vi "Drive Controller.vi"(8 "error in":errorcluster) -> ()   [LabVIEW 2023]
doc: "This VI executes continuously carrying out the current operation and responding to updates or new operation requests. It will often contain the timing or control code that is difficult to place directly in TeleOp. This VI generally opens all sensors and motors and isolates the rest of the robot code from knowing implementation details of how the operations are carried out."
uses:
  Drive Operations.ctl
  bordeaux-pathinator/Bordeaux/Types/Segment Type.ctl
  Drive Setpoints.ctl
  swerve/Type Definitions/Data/Robot Velocities.ctl
  <vilib>/Rock Robotics/WPI/ThirdParty/REV Robotics/REVLib/Typedef/Spark MAX Control Type.ctl
  <vilib>/Rock Robotics/WPI/DriverStation/WPI_DriverStationRobotMode2.ctl
  e7fadf63-5109-474c-80f5-604bef1b4eb3.vi
  80b923c8-6b82-42f9-a8cd-acddf0fa8107.vi
  Framework/Robot Global Data.vi
  <vilib>/Rock Robotics/Network Tables/NT Write String.vi
  <vilib>/Rock Robotics/Network Tables/NT Read Numeric Array.vi
  <vilib>/Rock Robotics/Network Tables/NT Read Number.vi
  <vilib>/Platform/TimedLoop/XDataNode/XDataNode.xnode
  <vilib>/Platform/TimedLoop/XDataNode/nitl_modes.ctl
  <vilib>/Platform/TimedLoop/XDataNode/XDNodeRunTimeDep.lvlib
  <vilib>/Platform/TimedLoop/XDataNode/wakeup.ctl
  <vilib>/Platform/TimedLoop/XDataNode/timing_clust.ctl
  <vilib>/ptbypt/NI_PtbyPt.lvlib
  <vilib>/Rock Robotics/WPI/ThirdParty/Phoenix-LabVIEW/Pigeon IMU/CTRE_PigeonIMU_GetYPR.vi
panel:
  in  "Y Setpoint":dbl=-1.5
  in  "Right PID Setpoint":dbl=0.545
  in  "Left PID Setpoint":dbl=-0.49
  in  "Freeze Align?":bool
  out "VMag Sum":dbl
  out "Enabled VMag":dbl[](graph)
  out "Sum Angle":dbl
  out "Sum Y":dbl
  out "Sum X":dbl
  out "Enabled Omega":dbl[](graph)=[-0.0]
  out "Enabled Y Velocity":dbl[](graph)
  out "Enabled X Velocity":dbl[](graph)
  out "Trajectory Velocity":dbl[](graph)
  out "Trajectory Data Compare":T2(array[cluster])
  out "Trajectory Data Out":T2(array[cluster])=[{"Segment Name"="Linear 0", "Type"=enum."Accel Straight", "Traj Pos Points"=[{"x"=-0.07702359916175033, "y"=-1.5597275539829196, "th"=0.3959786593914032}], "Traj Vel Points"=[{"V"=0.0, "Omega"=-0.0, "V vector"={"y"=-0.0, "x"=0.0}}], "Accel Index"=0, "Decel Index"=1}, {"Segment Name"="", "Type"=enum."Accel Straight", "Traj Pos Points"=[], "Traj Vel Points"=[], "Accel Index"=0, "Decel Index"=0}]
  in  "PID enabled":bool=TRUE
  out "Trapezoid Profile":dbl[](graph)
  out "Weird Aligning Code?":string
  in  "Go Up?":i32
  in  "Int per ft":dbl=0.75
  in  "PID gains":T3={"proportional gain (Kp)"=1.5, "integral time (Ki)"=0.075, "derivative time (Kd)"=0.0} {"derivative time (Kd)" format="%.3f"; "integral time (Ki)" format="%.3f"; "proportional gain (Kp)" format="%.3f"}
  out "PID Out":dbl=0.10498956284304024
  out "Waveform Chart":cluster{dbl, "Right X Setpoint":dbl}(graph)={-0.574331443611901, "Right X Setpoint"=-0.559167}
  in  "Operation":T4
  in  "Auto PID Constants":T5={"P Gain"=0.09, "I Gain"=0.0, "D Gain"=0.0, "F Gain"=0.08, "I Zone"=0.0, "Min Output"=-1.0, "Max Output"=1.0}
  in  "Immediate PID Constants":T5={"P Gain"=0.09, "I Gain"=0.0, "D Gain"=0.0, "F Gain"=0.08, "I Zone"=0.0, "Min Output"=-1.0, "Max Output"=1.0}
  out "Waveform Chart":cluster{"Numeric":dbl, "Numeric":dbl}(graph)
  in  "Period":i32=26
  in  "Acceleration Max":dbl=3.0
  in  "Velocity Max":dbl=6.0
  in  "Left X Setpoint":dbl=-0.609167
  in  "Left Y Setpoint":dbl
  in  "Right Y Setpoint":dbl
  in  "Right X Setpoint":dbl=0.559167
  in  "Deadband":T6={"Angle (deg)"=3.0, "X (ft)"=0.1, "Y (ft)"=0.125}
  in  "Drive Controller Diagnostics":T7(tab)
  out "Swerve Visualizer":cluster{dbl[], dbl[]}[](graph)
  out "Pod Comparisons (Diff -> Setpoint - Actual)":T8
  out "(Calibration) Steering Angles":T9={"Left Front"=134.8391571044922, "Left Back"=135.21200561523438, "Right Front"=135.20999145507812, "Right Back"=-44.576202392578125}
  out "Current\nCmd":string="Started at  21:02:15.312\nDefault: Reserve,  Vx 0.0, Vy 0.0, W 0.000000"
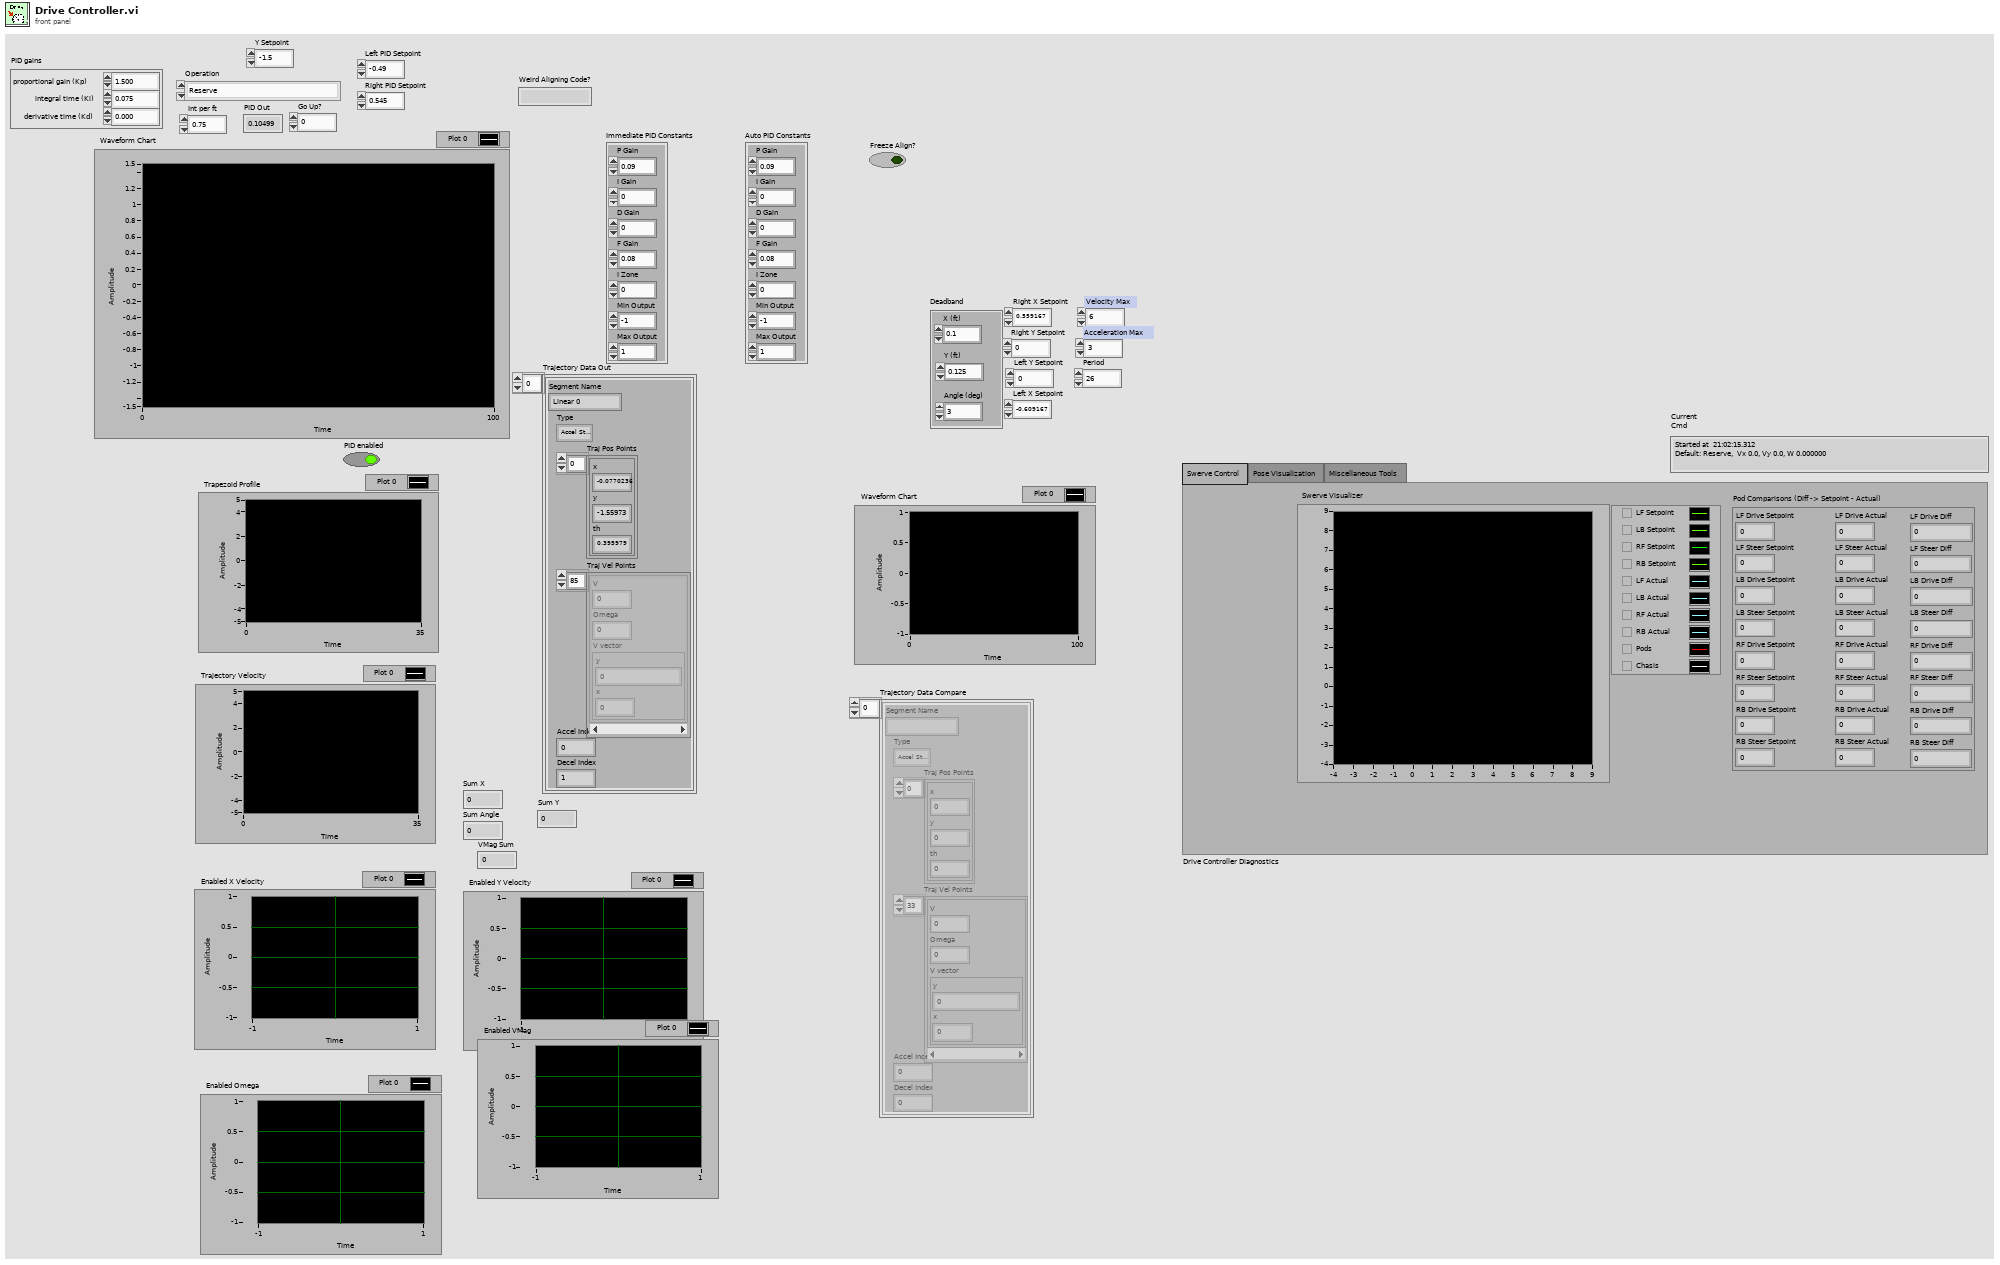
[diagram p1: front panel]
types:
  T1 = typedef "Segment Type.ctl" = enum16{"Accel Straight", "Const Straight", "Blend", "Circle", "Bezier"}
  T2 = cluster{"Segment Name":string, "Type":T1, "Traj Pos Points":cluster{"x":dbl, "y":dbl, "th":dbl}[], "Traj Vel Points":cluster{"V":dbl, "Omega":dbl, "V vector":cluster{"y":dbl, "x":dbl}}[], "Accel Index":i32, "Decel Index":i32}[]
  T3 = cluster{"proportional gain (Kp)":dbl, "integral time (Ki)":dbl, "derivative time (Kd)":dbl}
  T4 = typedef "Drive Operations.ctl" = enum16{"Reserve", "Read Current", "Immediate", "Calibrate", "Reef Align", "Auto"}
  T5 = cluster{"P Gain":dbl, "I Gain":dbl, "D Gain":dbl, "F Gain":dbl, "I Zone":dbl, "Min Output":dbl, "Max Output":dbl}
  T6 = cluster{"Angle (deg)":dbl, "X (ft)":dbl, "Y (ft)":dbl}
  T7 = enum32{"Swerve Control", "Pose Visualization", "Miscellaneous Tools"}
  T8 = cluster{"LF Drive Setpoint":dbl, "LF Steer Setpoint":dbl, "LB Drive Setpoint":dbl, "LB Steer Setpoint":dbl, "RF Drive Setpoint":dbl, "RF Steer Setpoint":dbl, "RB Drive Setpoint":dbl, "RB Steer Setpoint":dbl, "LF Drive Actual":dbl, "LF Steer Actual":dbl, "LB Drive Actual":dbl, "LB Steer Actual":dbl, "RF Drive Actual":dbl, "RF Steer Actual":dbl, "RB Drive Actual":dbl, "RB Steer Actual":dbl, "LF Drive Diff":dbl, "LF Steer Diff":dbl, "LB Drive Diff":dbl, "LB Steer Diff":dbl, "RF Drive Diff":dbl, "RF Steer Diff":dbl, "RB Drive Diff":dbl, "RB Steer Diff":dbl}
  T9 = cluster{"Left Front":dbl, "Left Back":dbl, "Right Front":dbl, "Right Back":dbl}
  T10 = typedef "Drive Setpoints.ctl" = cluster{"Operation":T4, "Robot Velocities":T11, "Auto Data":cluster{"Auto Velocities":T11[], "Auto Positions":cluster{"x":dbl, "y":dbl, "th":dbl}[], "Auto Commands":cluster{dbl, "Command out":cluster{"Name":string, "vi reference":refnum<vi>, i32[], variant[]}}[], "Zero Velocity?":bool[]}, "Left side":bool, "Angle Align":bool, "Tag ID":i32}
  T11 = typedef "Robot Velocities.ctl" = cluster{"X Velocity":dbl, "Y Velocity":dbl, "Rotational \nVelocity":dbl}
  T12 = typedef "(NEO-NEO-ThroughBore-Pigeon2) Swerve.ctl" = cluster{"Drive Motors (NEO)":T13, "Steer Motors (NEO)":T13, "Pigeon2":T19, "Radii (ft)":T21}
  T13 = typedef "(NEO & NEO 550) 4 Motor Set.ctl" = cluster{"Left Front":T14, "Left Back":T14, "Right Front":T14, "Right Back":T14}
  T14 = typedef "WPI_MotorControlDeviceRef.ctl" = cluster{"DeviceStatus":errorcluster, "Type":T15, "PWM":cluster{"PWM Channel":T16, "DeadBand":T17}, "CAN":cluster{"Device Number":u8, "SetOutput VI Ref":variant, "GetOutput VI Ref":variant, "Enable VI Ref":variant, "Disable VI Ref":variant, "Data":variant}, "Invert":bool, "DIO PWM":cluster{"PWM \"Enable\" Channel":T16, "DIOChannel":T18, "PWM Rate":dbl}}
  T15 = typedef "WPI_MotorControlType.ctl" = enum16{"PWM", "CAN", "DIO PWM"}
  T16 = typedef "FPGA_DIOPWMChannel.ctl" = enum8{"PWM 0", "PWM 1", "PWM 2", "PWM 3", "PWM 4", "PWM 5", "PWM 6", "PWM 7", "PWM 8", "PWM 9", "PWM MXP 0", "PWM MXP 1", "PWM MXP 2", "PWM MXP 3", "PWM MXP 4", "PWM MXP 5", "PWM MXP 6", "PWM MXP 7", "PWM MXP 8", "PWM MXP 9", "Invalid"}
  T17 = typedef "WPI_PWMDeadband.ctl" = cluster{"Name":string, "maxPositivePwm":i32, "minPositivePwm":i32, "centerPwm":i32, "maxNegativePwm":i32, "minNegativePwm":i32, "angularRange":u16}
  T18 = typedef "FPGA_DIOChannel.ctl" = enum8{"DIO 0", "DIO 1", "DIO 2", "DIO 3", "DIO 4", "DIO 5", "DIO 6", "DIO 7", "DIO 8", "DIO 9", "DIO MXP 0", "DIO MXP 1", "DIO MXP 2", "DIO MXP 3", "DIO MXP 4", "DIO MXP 5", "DIO MXP 6", "DIO MXP 7", "DIO MXP 8", "DIO MXP 9", "DIO MXP 10", "DIO MXP 11", "DIO MXP 12", "DIO MXP 13", "DIO MXP 14", "DIO MXP 15", "SPI Port CS1", "SPI Port CS2", "SPI Port CS3", "SPI Port MISO", "SPI Port MOSI", "Invalid"}
  T19 = typedef "CTRE_PigeonIMU_DeviceRef.ctl" = cluster{"DeviceStatus":errorcluster, "Device Number":u8, "Type":T20, "Device ID":u32, "Handle":u64, "UsageFrame":u32, "Library Path":path}
  T20 = typedef "CTRE_PigeonIMU_ConnectionType.ctl" = u32
  T21 = typedef "Pod Positions.ctl" = cluster{"Left Front Position":dbl[], "Left Back Position":dbl[], "Right Front Position":dbl[], "Right Back Position":dbl[]}
  T22 = typedef "Command Status Info.ctl" = cluster{"Name":string, "Status":T23, "notifier out":T24}
  T23 = typedef "Completion Status.ctl" = enum16{"Successful", "Aborted", "Incomplete"}
  T24 = typedef "Completion Notifier.ctl" = refnum<notifier>
  T25 = cluster{"SubSystem Data":T10, cluster{"Start Time (ms)":u32, "Iterations":i32}, cluster{"Command Info":T22, "Description":string, "Default Command":T10, "queue out":refnum<queue>, "Subsystem Name":string}}
  T26 = typedef "Spark MAX Control Type.ctl" = enum16{"Percent VBus", "Voltage", "Velocity", "Position", "Smart Motion", "Current", "Smart Velocity", "MAXMotion Position", "MAXMotion Velocity"}
  T27 = typedef "WPI_DriverStationRobotMode2.ctl" = enum16{"Autonomous Disabled", "Autonomous Enabled", "Teleop Disabled", "Teleop Enabled", "Disconnected", "Finish", "Test Disabled", "Test Enabled", "Emergency Stopped"}
  T28 = typedef "XDNodeRunTimeDep.lvlib/timing_clust.ctl" = cluster{"Expected End [f-1]":u64, "Actual End [f-1]":u64, "Finished Late? [f-1]":bool, "Expected End [i-1]":u64, "Actual End [i-1]":u64, "Finished Late? [i-1]":bool, "Expected Start [i]":u64, "Actual Start [i]":u64, "Expected Start [f]":u64, "Actual Start [f]":u64, "Source Name":string, "Structure Name":string, "Period":i64, "Deadline":i64, "Offset":i64, "Start":i64, "Priority":i32, "Timeout":i32, "Mode":T29, "Wakeup Reason":T30, "Error":errorcluster, "Source Type":string, "Secondary Source Type":string, "Global End Time":u64, "Global Start Time":u64, "Frame Duration":u64, "Iteration Duration":u64, "Assigned CPU":i32, "I/O Scan Engine Mode":u32}
  T29 = typedef "XDNodeRunTimeDep.lvlib/nitl_modes.ctl" = enum32{"No Change", "Process missed periods, maintain original phase", "Discard missed periods, maintain original phase", "Process missed periods, ignore original phase", "Discard missed periods, ignore original phase"}
  T30 = typedef "XDNodeRunTimeDep.lvlib/wakeup.ctl" = enum32{"Normal", "Aborted", "Asynchronous wakeup", "Timing source error", "Timed loop error", "Timeout"}
  T31 = cluster{"Auto Velocities":T11[], "Auto Positions":cluster{"x":dbl, "y":dbl, "th":dbl}[], "Auto Commands":cluster{dbl, "Command out":cluster{"Name":string, "vi reference":refnum<vi>, i32[], variant[]}}[], "Zero Velocity?":bool[]}
  T32 = cluster{"Field Centric":bool, "Reef Centric":bool}
  T33 = typedef "Pod Setpoints.ctl" = cluster{"Left Front":cluster{"Velocity":dbl, "Theta":dbl}, "Left Back":cluster{"Velocity":dbl, "Theta":dbl}, "Right Front":cluster{"Velocity":dbl, "Theta":dbl}, "Right Back":cluster{"Velocity":dbl, "Theta":dbl}}
  T34 = cluster{"Left X Setpoint":dbl, "Left Y Setpoint":dbl}
  T35 = cluster{"Right X Setpoint":dbl, "Right Y Setpoint":dbl}
  T36 = cluster{"Segment Name":string, "Type":T1, "Traj Pos Points":cluster{"x":dbl, "y":dbl, "th":dbl}[], "Traj Vel Points":cluster{"V":dbl, "Omega":dbl, "V vector":cluster{"y":dbl, "x":dbl}}[], "Accel Index":i32, "Decel Index":i32}
  T37 = cluster{"V":dbl, "Omega":dbl, "V vector":cluster{"y":dbl, "x":dbl}}[]
  T38 = cluster{"Filtered x":dbl, "Right X Setpoint":dbl}
  T39 = cluster{"Right X Setpoint":dbl, "Y Setpoint":dbl, dbl}
  T40 = cluster{"SubSystem Data":T10, cluster{"Start Time (ms)":u32, "Iterations":i32}, "Default Command Arguments":cluster{"Command Info":T22, "Description":string, "Default Command":T10, "queue out":refnum<queue>, "Subsystem Name":string}}
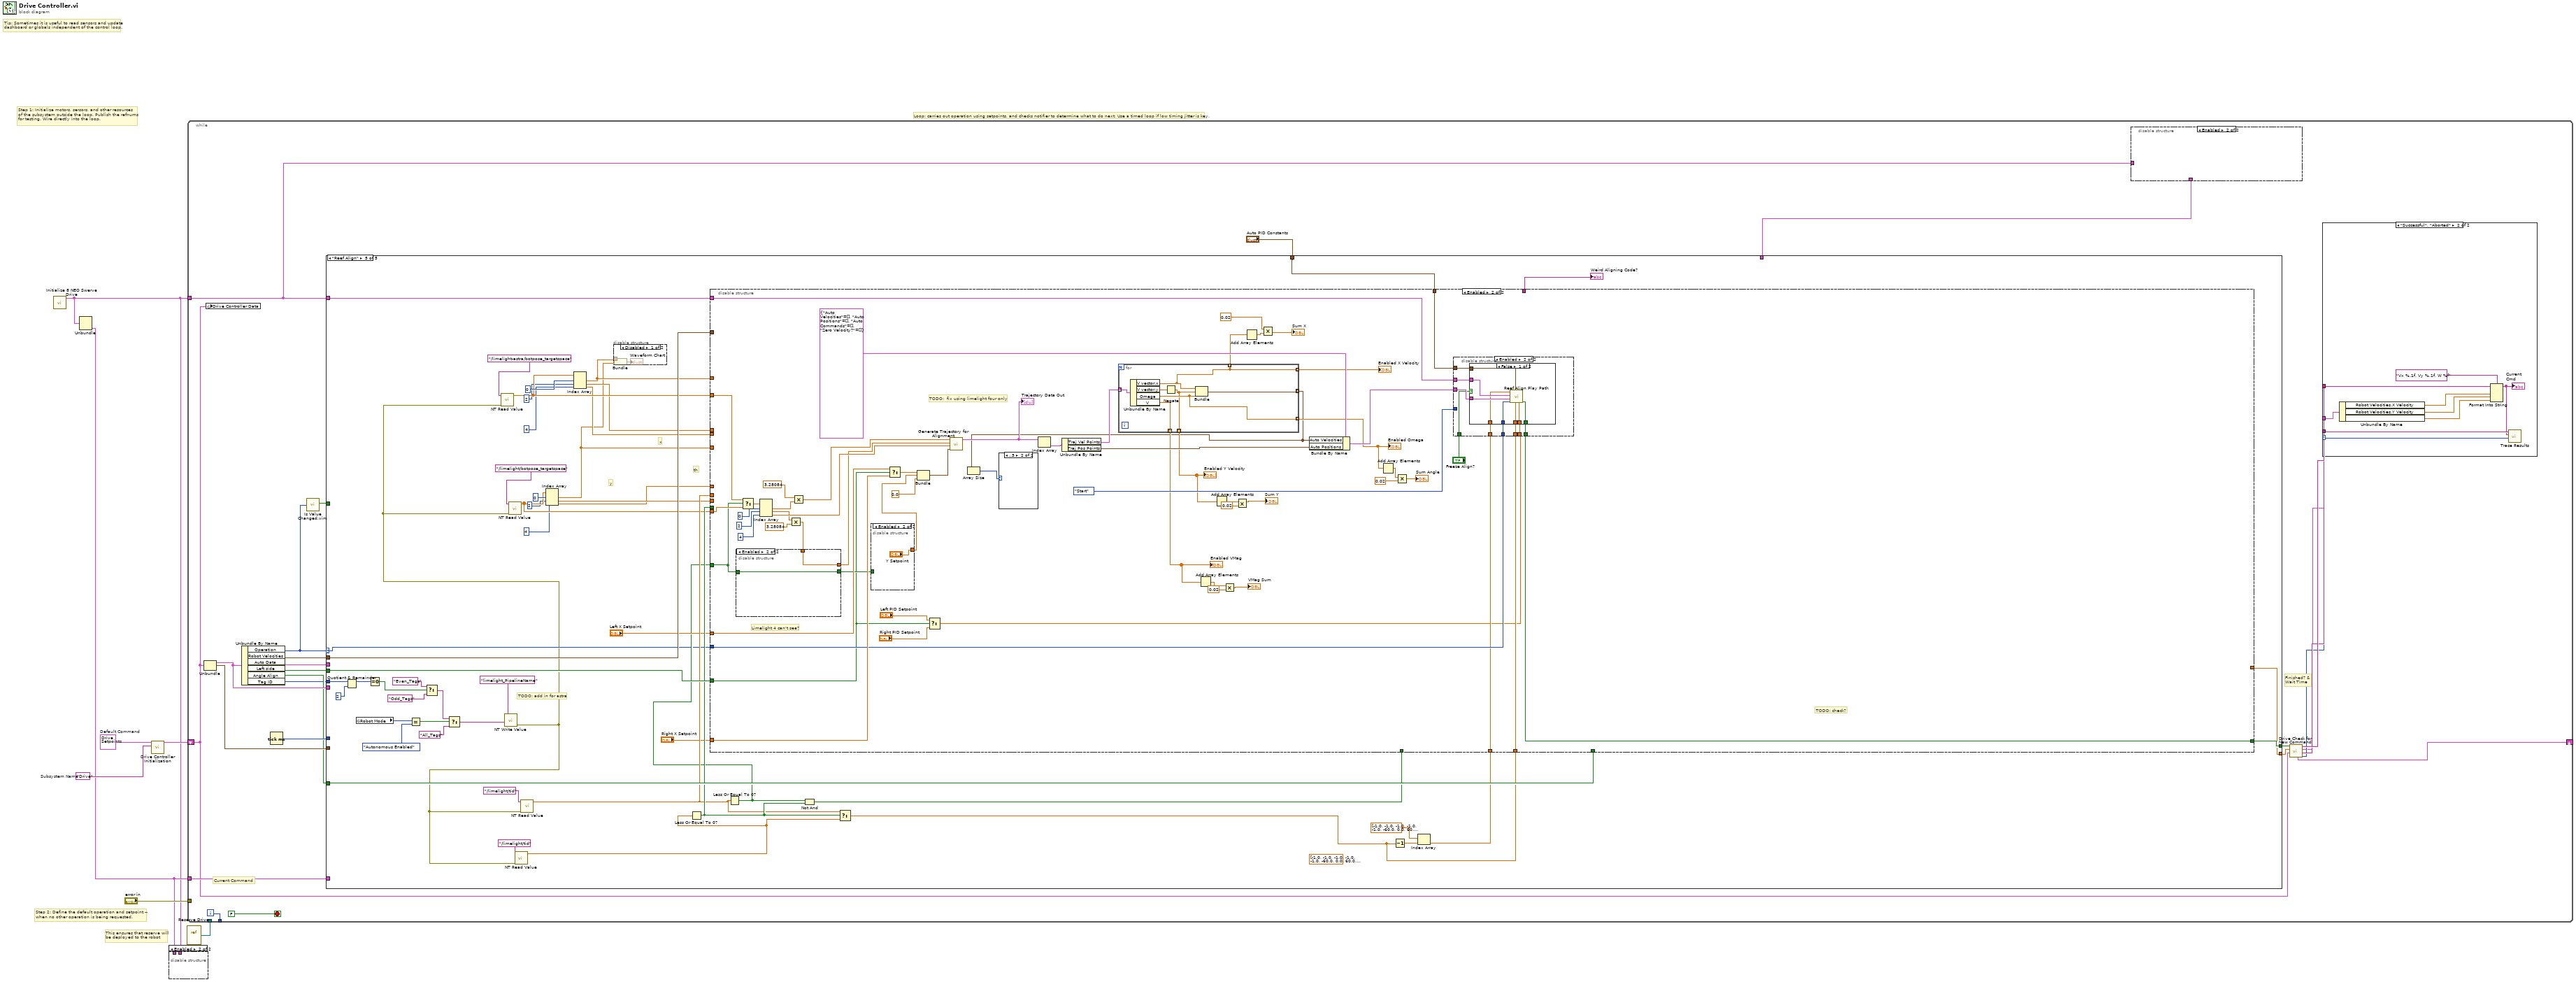
[diagram p0: block diagram]
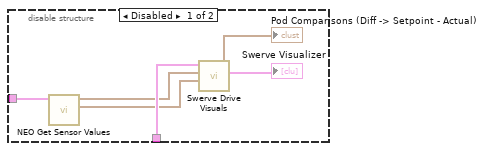
[diagram p2: hidden frame]
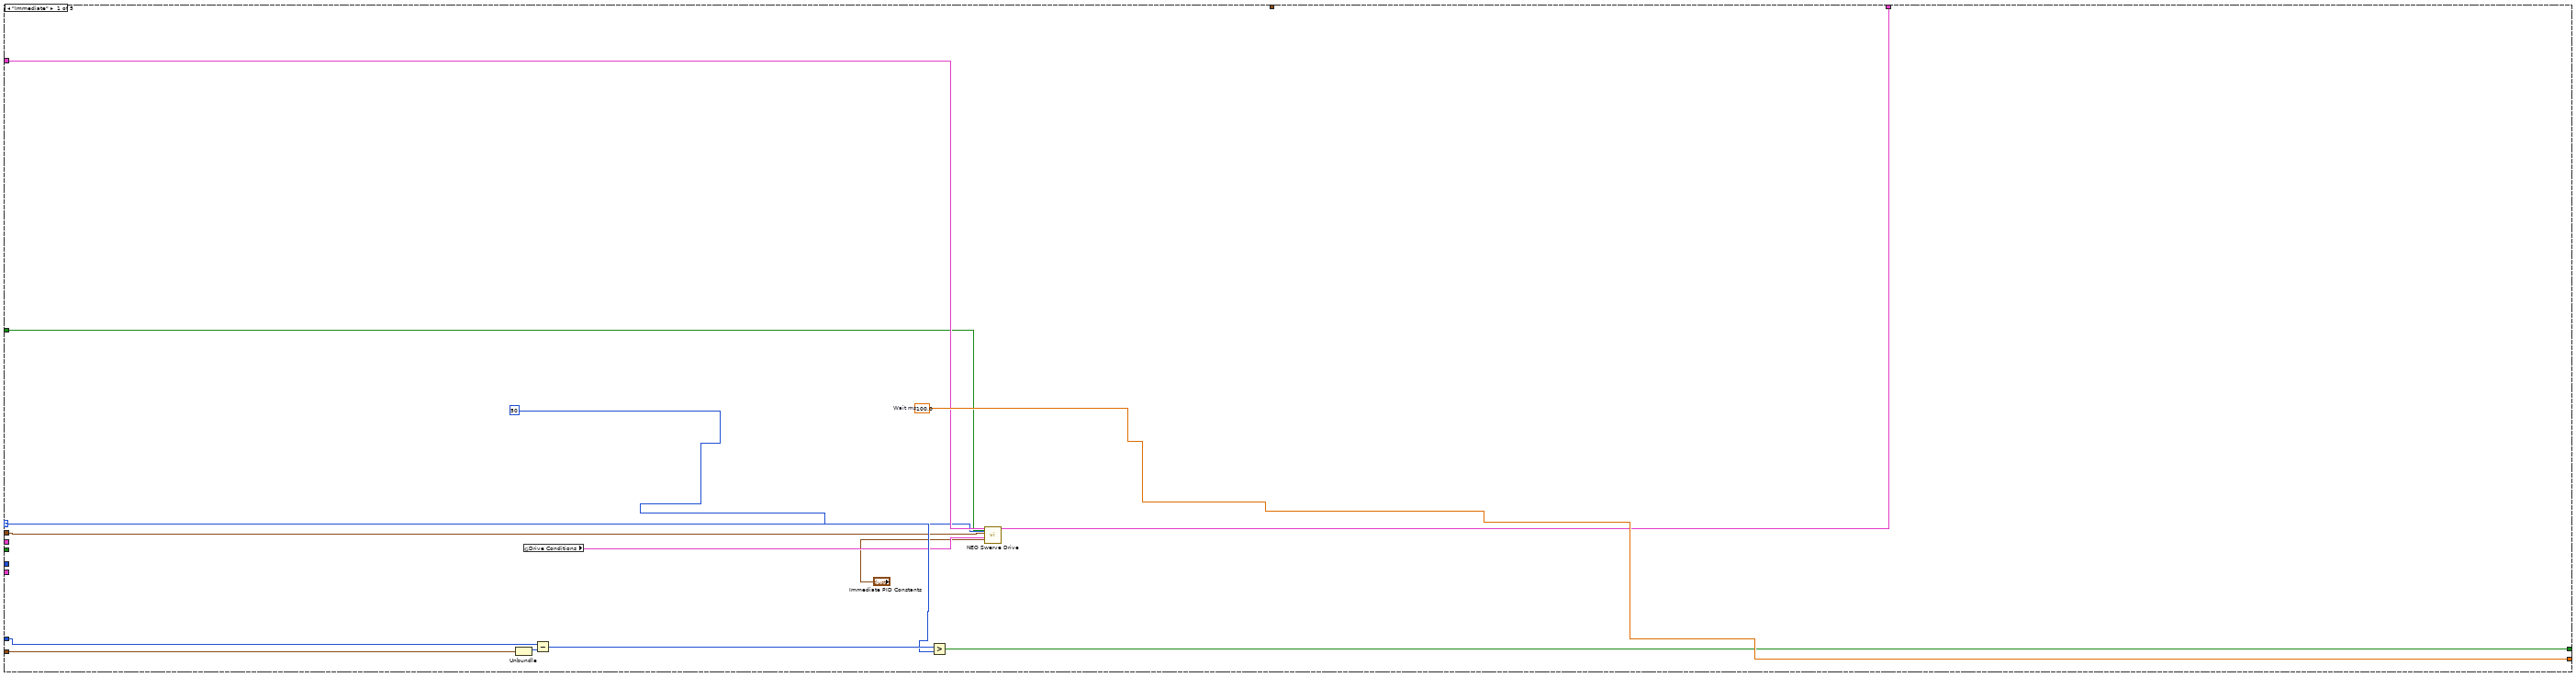
[diagram p3: hidden frame]
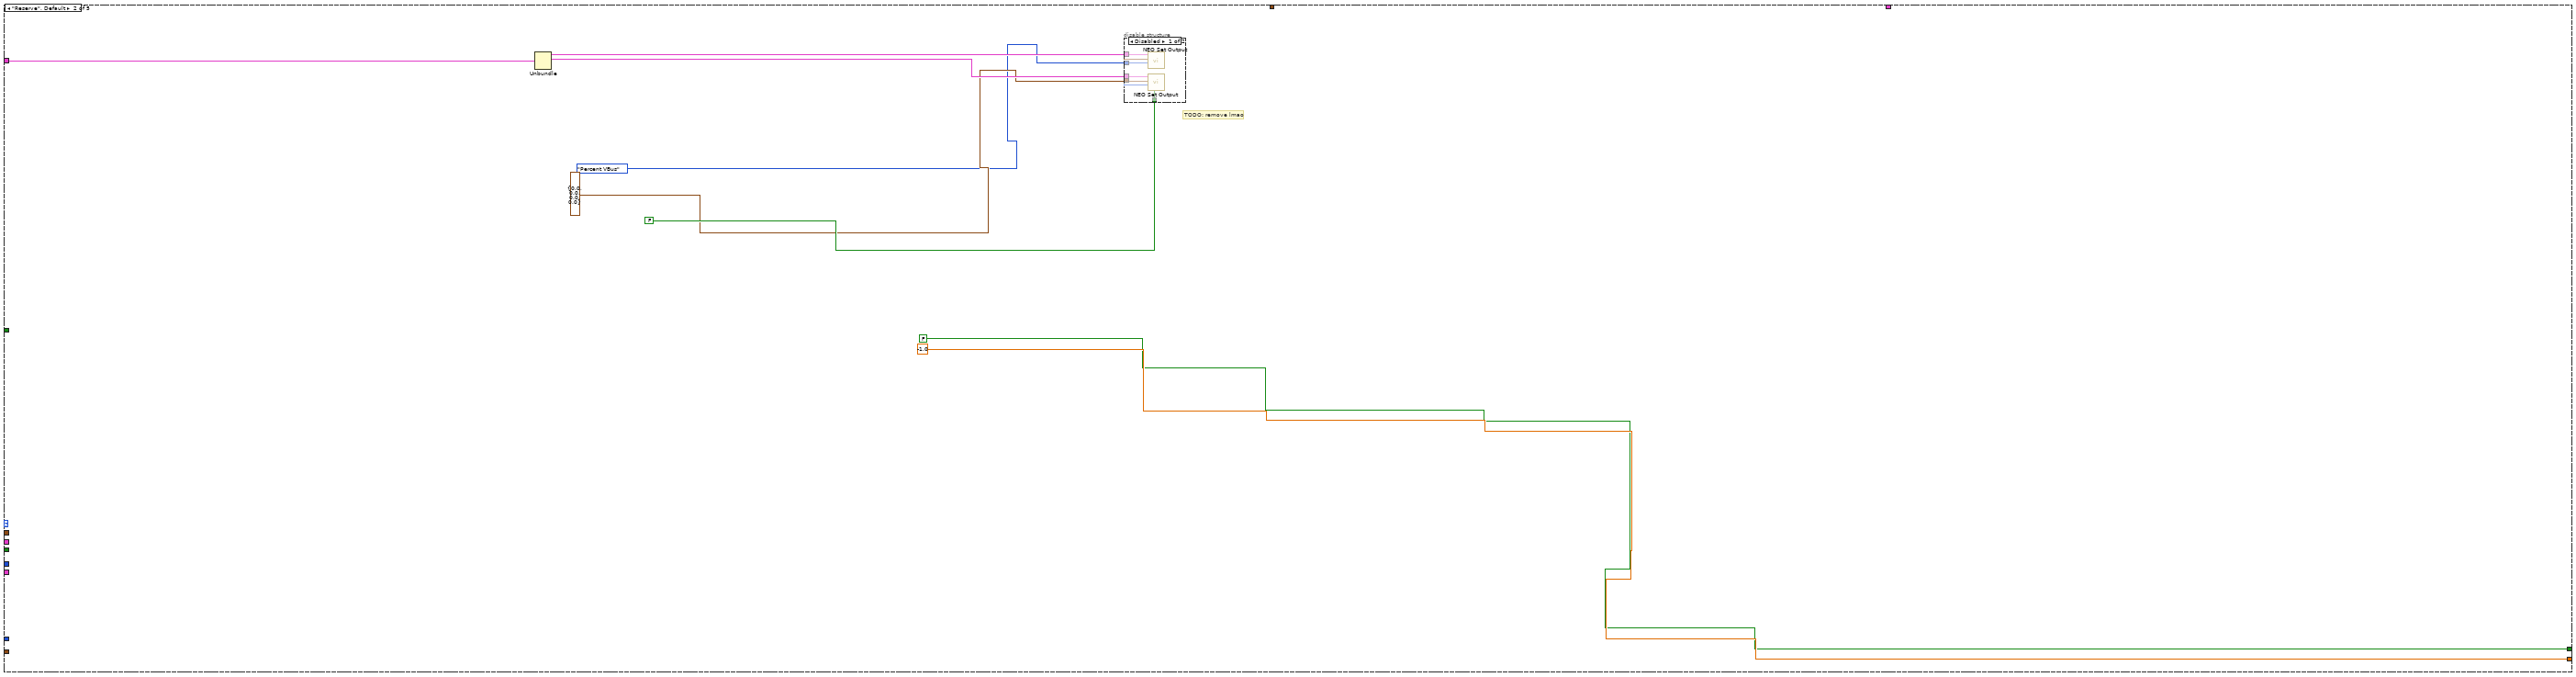
[diagram p4: hidden frame]
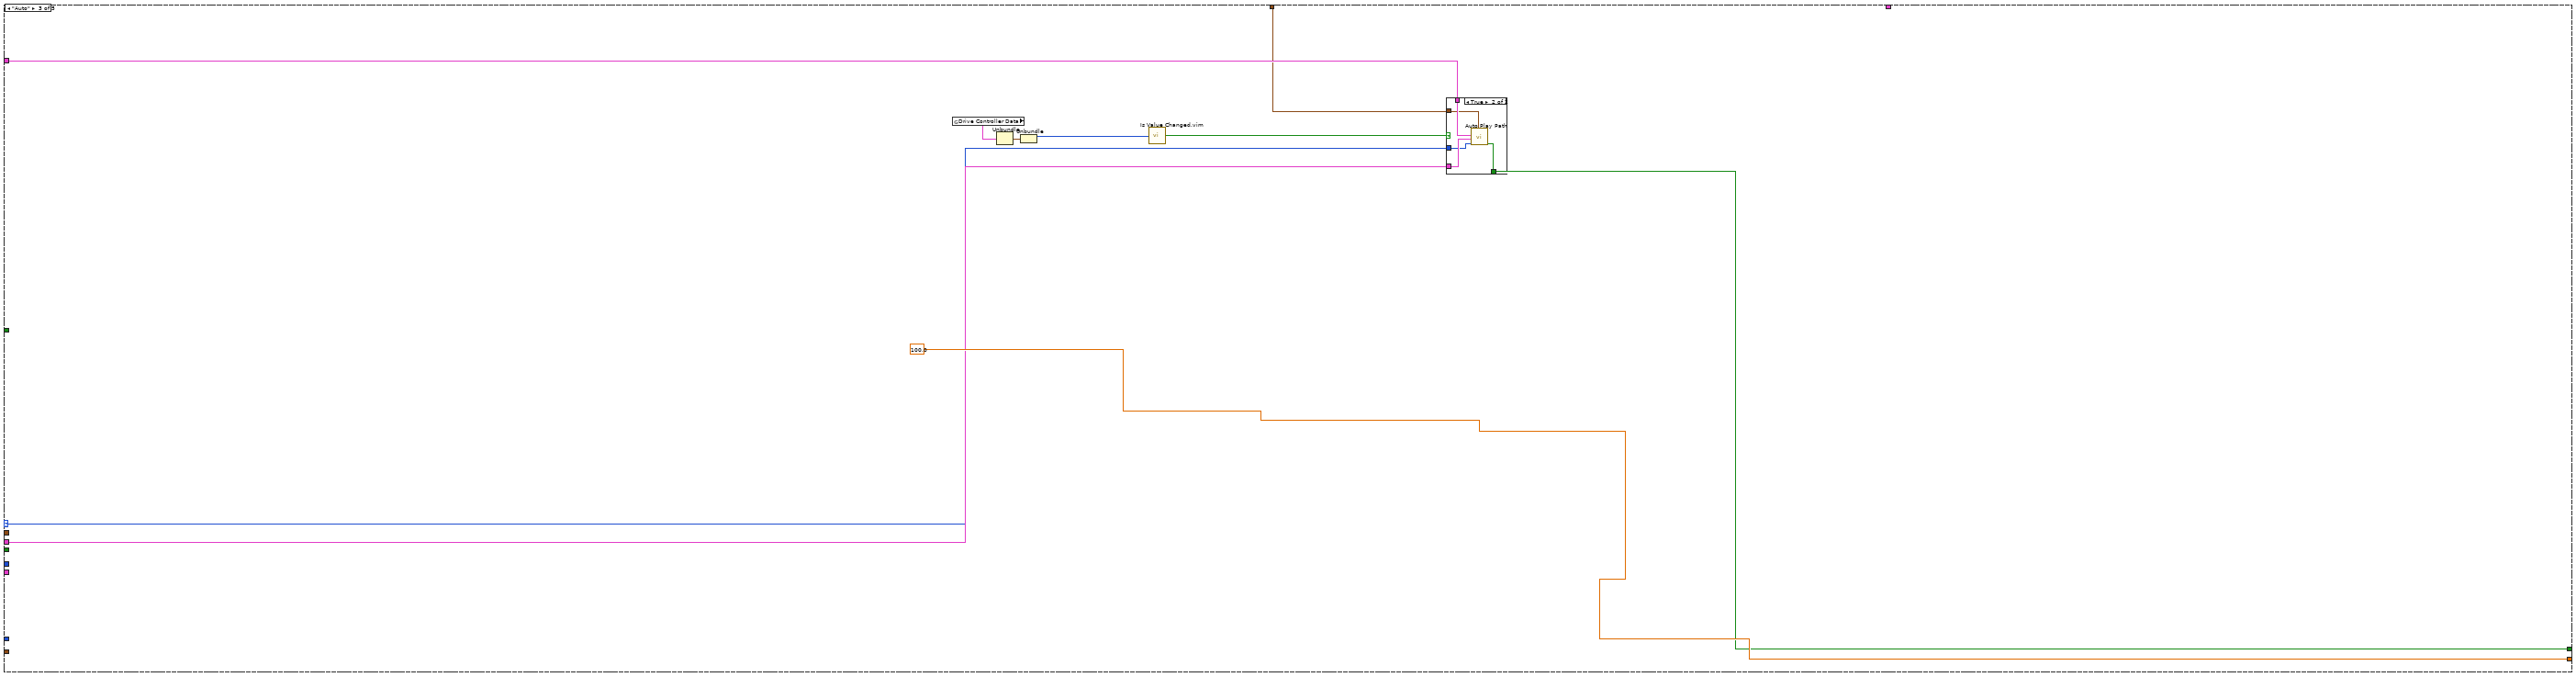
[diagram p6: hidden frame]
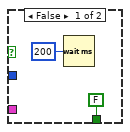
[diagram p7: hidden frame]
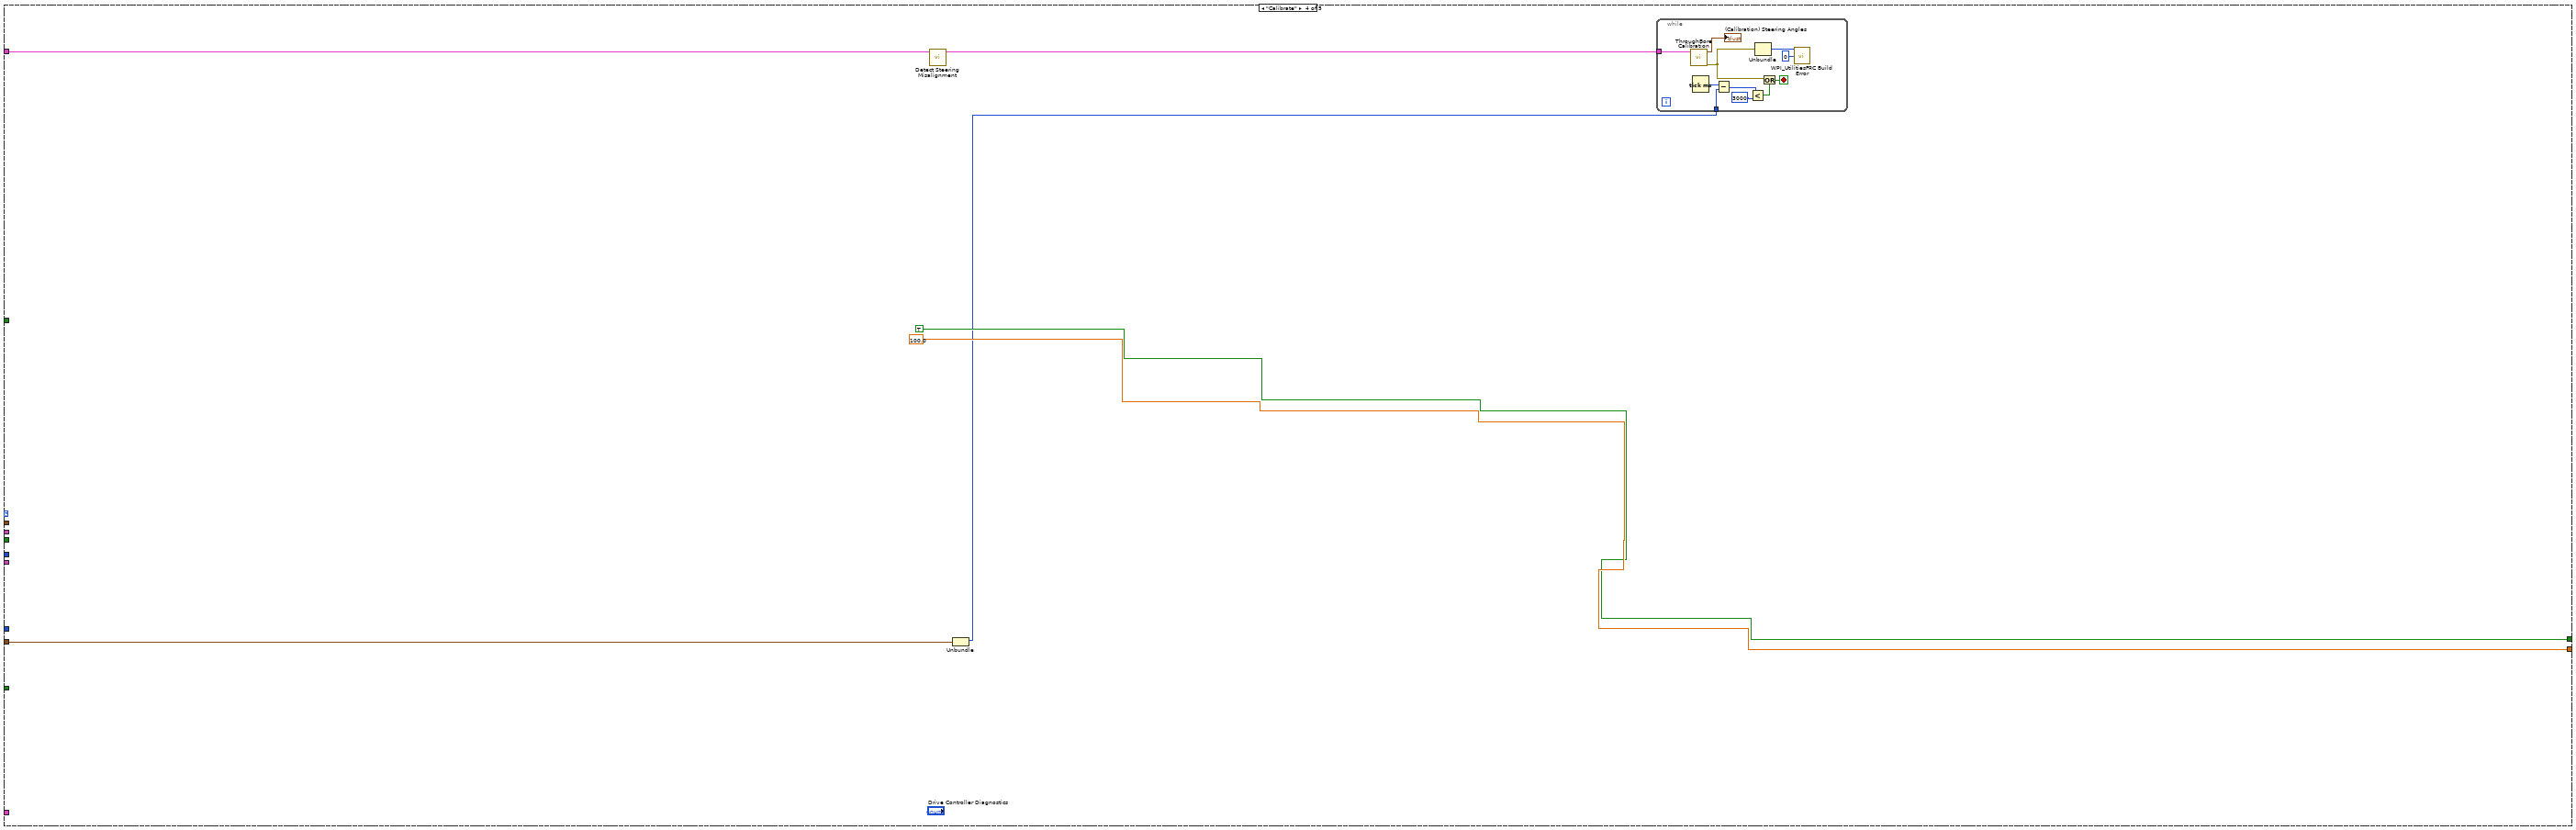
[diagram p8: hidden frame]
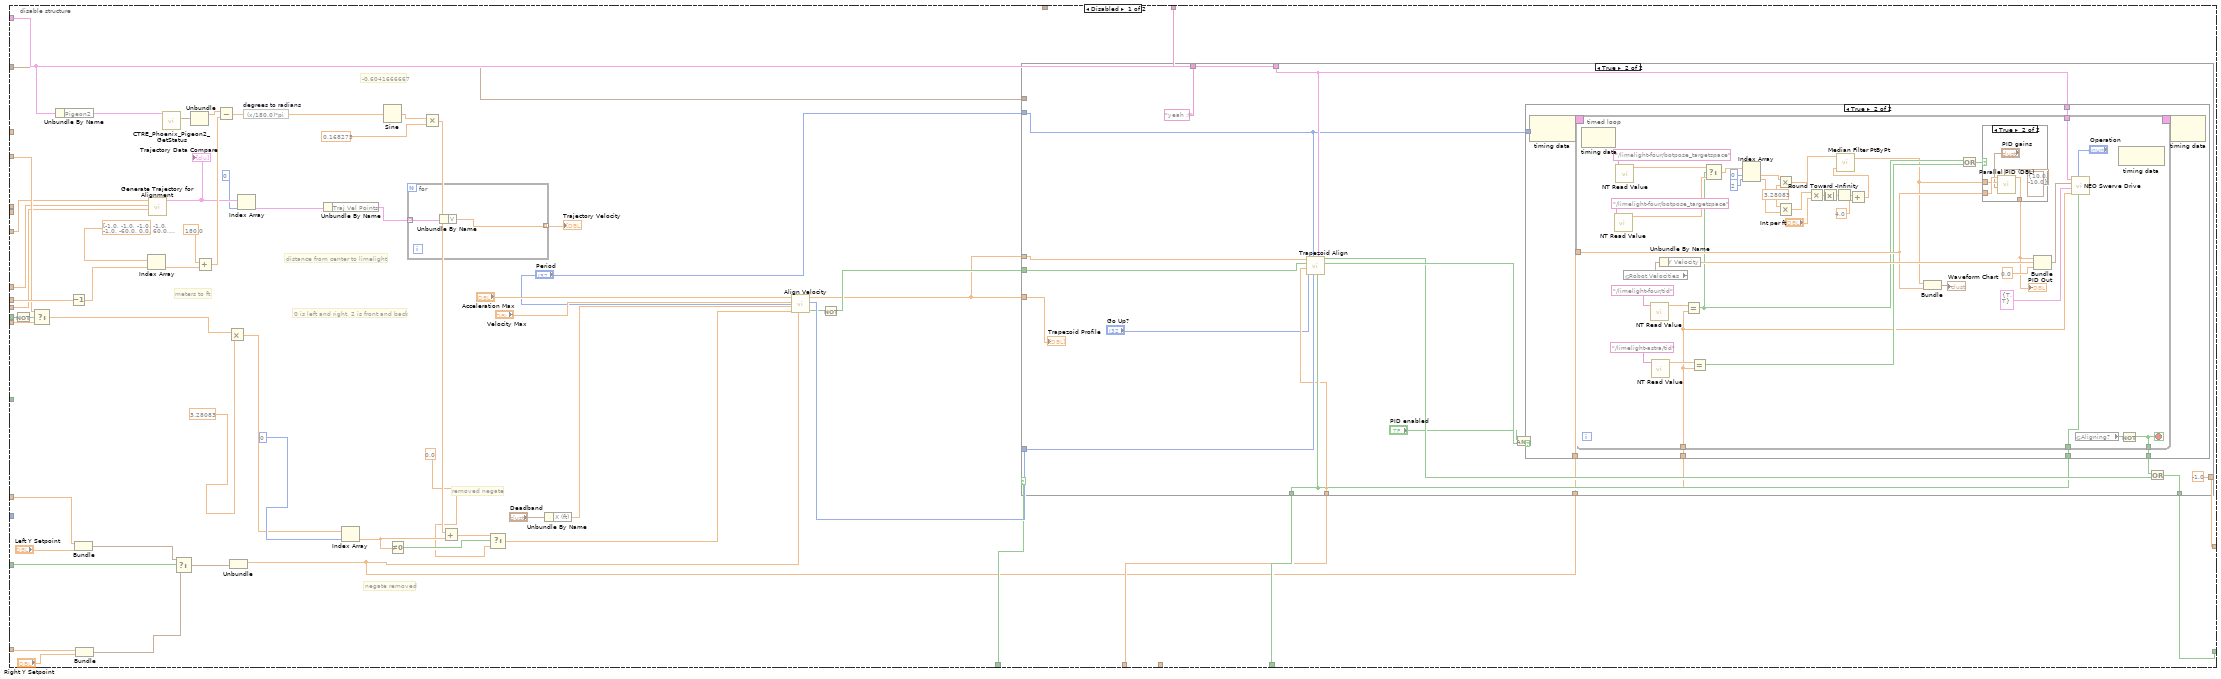
[diagram p10: hidden frame]
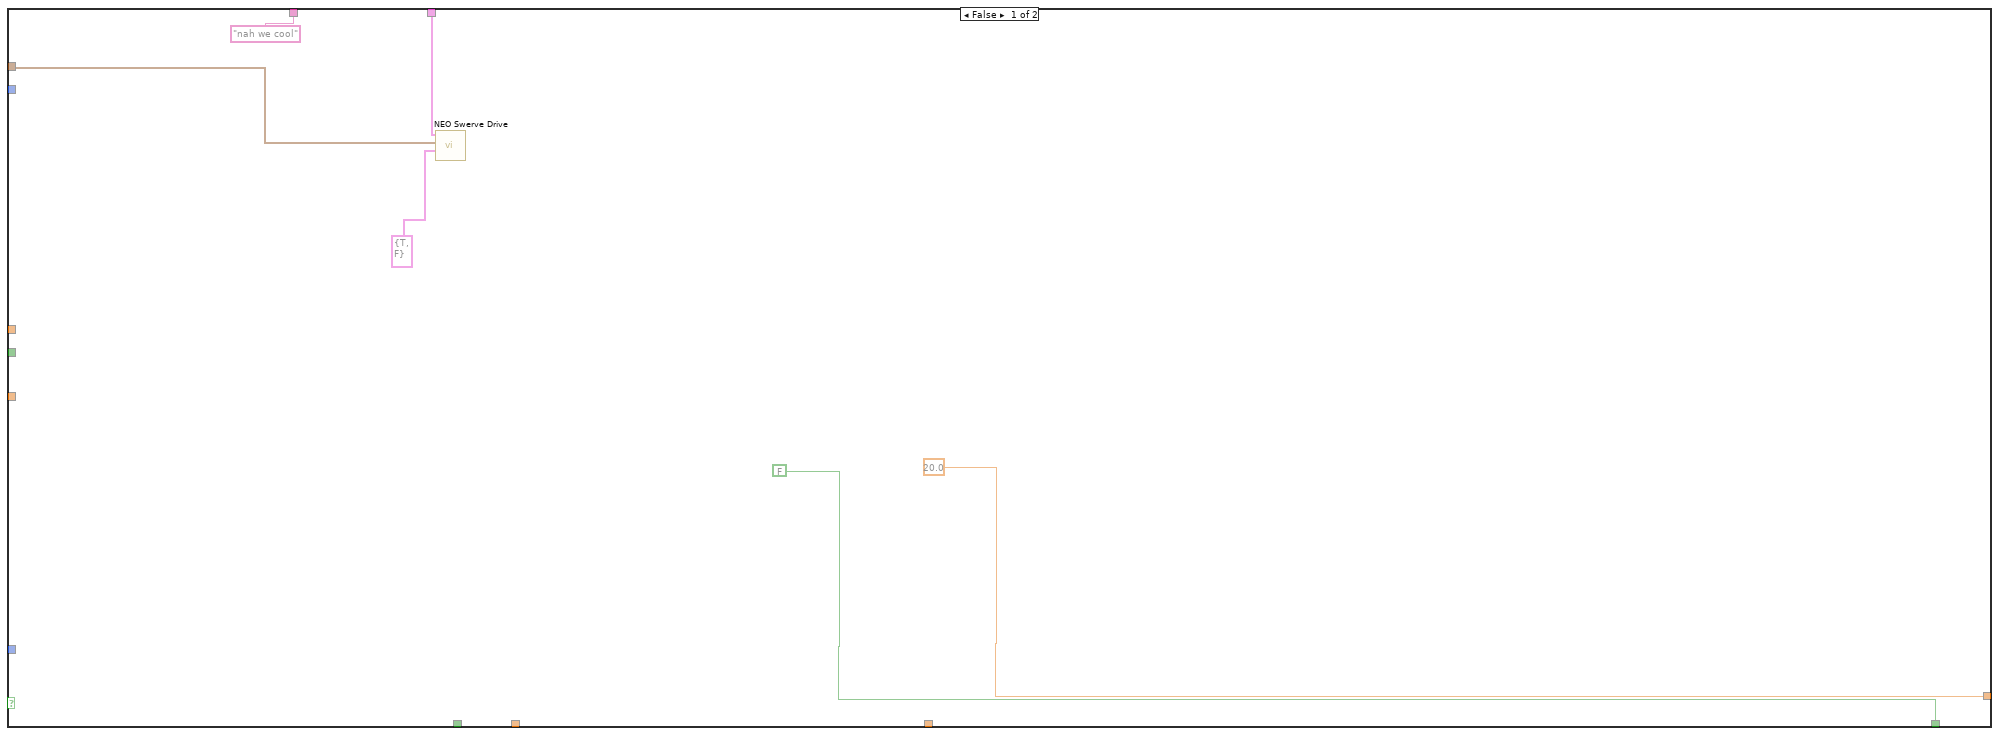
[diagram p11: hidden frame]
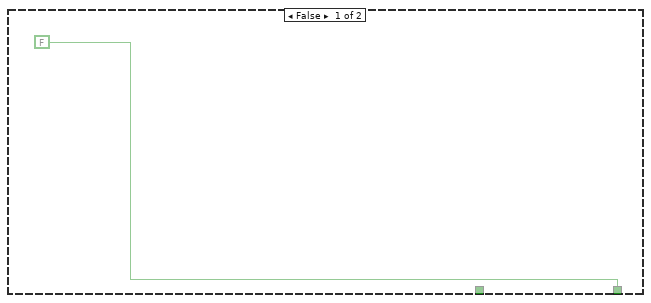
[diagram p12: hidden frame]
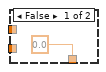
[diagram p13: hidden frame]
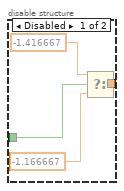
[diagram p15: hidden frame]
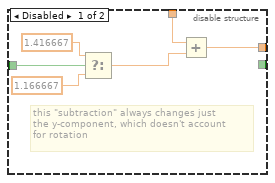
[diagram p16: hidden frame]
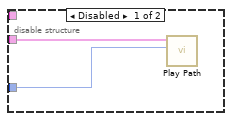
[diagram p17: hidden frame]
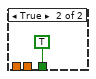
[diagram p18: hidden frame]
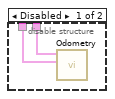
[diagram p20: hidden frame]
diagram:
  w3 = T10 {"Operation"=enum."Reserve", "Robot Velocities"={"X Velocity"=0.0, "Y Velocity"=0.0, "Rotational \nVelocity"=0.0}, "Auto Data"={"Auto Velocities"=[], "Auto Positions"=[], "Auto Commands"=[], "Zero Velocity?"=[]}, "Left side"=FALSE, "Angle Align"=FALSE, "Tag ID"=0}  # Default Command
  w7 = "Drive"  # Subsystem Name
  # "This ensures that reserve will\nbe deployed to the robot"
  # "Step 2: Define the default operation and setpoint --\nwhen no other operation is being requested."
  # "Step 1: Initialize motors, sersors, and other resources\nof the subsystem outside the loop. Publish the refnums\nfor testing. Wire directly into the loop."
  # "Loop: carries out operation using setpoints, and checks notifier to determine what to do next. Use a timed loop if low timing jitter is key."
  # "Tip: Sometimes it is useful to read sensors and update\ndashboard or globals independent of the control loop."
  n1 = call "Initialize 8 NEO Swerve Drive.vi"() -> ("Motors"=w1:T12)  [unwired: 10 in, 1 out]
  n2 = Unbundle(w1) -> ("Radii (ft)"=w2:T21)  [unwired: 3 out]
  n3 = call "Drive Controller Initialization.vi"("Subsystem Name"=w7, "Default Command"=w3) -> ("Current Command"=w5:T25)  [unwired: 9 in]
  n4 = disable-structure shown="Enabled" {
    disable-tunnel: w2 -> [w9 _]
    disable-tunnel: w1 -> [w8 _]
    frame Disabled {
      n5 = call "Odometry.vi"("Radii (ft)"=w9, "Motors"=w8) -> ()  [unwired: 10 in]
    }
    frame Enabled {
    }
  }
  n6 = vi-ref "Reserve Drive.vi"() -> (w4:refnum<vi>)
  n7 = while {
    shift-right: [w25] -> _
    shift-left: w5 -> [w16]
    tunnel: [w32] -> _
    tunnel: "error in" -> [_]
    tunnel: w4 -> [_]
    tunnel: w1 -> [w23]
    tunnel: w2 -> [w26]
    i -> [w32]
    stop <- FALSE stop-if-true
    # "Current Command"
    # "Finished? &\nWait Time"
    n8 = Unbundle(w16) -> ("SubSystem Data"=w19:T10, w17:cluster{"Start Time (ms)":u32, "Iterations":i32})  [unwired: 1 out]
    n9 = global write "Robot Global Data.vi" "Drive Controller Data"(w16) -> ()
    n10 = Unbundle By Name(w19) -> ("Operation"=w13:T4, "Robot Velocities"=w27:T11, "Auto Data"=w22:T31, "Left side"=w15:bool, "Angle Align"=w14:bool, "Tag ID"=w10:i32)
    n11 = Tick Count (ms)() -> (millisecond timer value=w18:u32)
    n12 = call "Is Value Changed.vim"("value"=w13) -> ("changed or first call?"=w12:bool)
    n13 = case shown="\"Reef Align\"" w13 {
      selector: w13 -> [w41 _ w69 _ w119]
      tunnel: [w53 -1.0 ("Infinite") 100.0 100.0 ("Infinite") w148] -> w31
      tunnel: [w48 FALSE ("ignore previous (F)") w68 TRUE ("ignore previous (F)") w152] -> w30
      tunnel: w17 -> [w52 _ _ w87 _]
      tunnel: w18 -> [w47 _ _ _ _]
      tunnel: w27 -> [w45 _ _ _ w149]
      tunnel: w23 -> [w43 w59 w76 w85 w151]
      tunnel: w26 -> [_ _ _ _ _]
      tunnel: [w46 _ _ _ _] -> w24
      tunnel: w19 -> [_ _ _ _ _]
      tunnel: w22 -> [_ _ w74 _ _]
      tunnel: w15 -> [_ _ _ _ w150]
      tunnel: w14 -> [_ _ _ _ w147]
      tunnel: w12 -> [w40 _ _ _ _]
      tunnel: "Auto PID Constants" -> [_ _ w67 _ w120]
      tunnel: w10 -> [_ _ _ _ w111]
      frame "Immediate" {
        w53 = 100.0  # Wait ms
        n14 = Unbundle(w52) -> ("Start Time (ms)"=w51:u32)  [unwired: 1 out]
        n15 = global read "Robot Global Data.vi" "Drive Conditions"() -> (w44:T32)
        n16 = Subtract(x=w47, y=w51) -> (x-y=w50:u32)
        n17 = Greater?(x=w50, y=u32 50) -> (0:w48:bool)
        n18 = call "NEO Swerve Drive.vi"("PID Constants"="Immediate PID Constants", "Configure?"=w40, "Operation"=w41, "Drive Conditions"=w44, "Robot Velocities"=w45, "Swerve Drive"=w43) -> ("Pod Setpoints (ft/s and deg)"=w46:T33)  [unwired: 5 in]
      }
      frame "Reserve", Default {
        # "TODO: remove lmao"
        n19 = Unbundle(w59) -> ("Drive Motors (NEO)"=w58:T13, "Steer Motors (NEO)"=w57:T13)  [unwired: 2 out]
        n20 = disable-structure shown="Disabled" {
          disable-tunnel: w58 -> [w66 _]
          disable-tunnel: w57 -> [w65 _]
          disable-tunnel: FALSE ("Add Angle Offsets?") -> [w64 _]
          disable-tunnel: T9 {"Left Front"=0.0, "Left Back"=0.0, "Right Front"=0.0, "Right Back"=0.0} ("Setpoints") -> [w63 _]
          disable-tunnel: Spark_MAX_Control_Type."Percent VBus" ("Reserve Control Mode") -> [w62 _]
          frame Disabled {
            n21 = call "NEO Set Output.vi"("Control Mode"=w62, "Setpoints"=w63, "Motors"=w66) -> ()  [unwired: 9 in]
            n22 = call "NEO Set Output.vi"("For Steer Motors?"=w64, "Control Mode"=w62, "Setpoints"=w63, "Motors"=w65) -> ()  [unwired: 8 in]
          }
          frame Enabled {
          }
        }
      }
      frame "Auto" {
        n23 = global read "Robot Global Data.vi" "Drive Controller Data"() -> (w73:T25)
        n24 = Unbundle(w73) -> (w72:cluster{"Start Time (ms)":u32, "Iterations":i32})  [unwired: 2 out]
        n25 = Unbundle(w72) -> ("Start Time (ms)"=w71:u32)  [unwired: 1 out]
        n26 = call "Is Value Changed.vim"("value"=w71) -> ("changed or first call?"=w70:bool)
        n27 = case shown="True" w70 {
          tunnel: w74 -> [_ w82]
          tunnel: w76 -> [_ w83]
          tunnel: w69 -> [_ w81]
          tunnel: [FALSE ("Auto Done?") w80] -> w68
          tunnel: w67 -> [_ w79]
          frame False {
            n28 = Wait (ms)(milliseconds to wait=u32 200) -> ()  [unwired: 1 out]
          }
          frame True {
            n29 = call "Auto Play Path.vi"("PID Constants"=w79, "Operation"=w81, "Auto Data"=w82, "Motors"=w83) -> ("Auto Done?"=w80:bool)  [unwired: 7 in]
          }
        }
      }
      frame "Calibrate" {
        n30 = call "Detect Steering Misalignment.vi"("Motors In"=w85) -> ("Motors Out"=w84:T12)  [unwired: 10 in]
        n31 = Unbundle(w87) -> ("Start Time (ms)"=w86:u32)  [unwired: 1 out]
        n32 = while {
          tunnel: w84 -> [w94]
          tunnel: w86 -> [w99]
          stop <- w100 stop-if-true
          n33 = call "ThroughBore Calibration.vi"("Motors"=w94) -> ("error out"=w91:errorcluster, "Steering Angles"=→"(Calibration) Steering Angles":cluster{"LF":dbl, "LB":dbl, "RF":dbl, "RB":dbl})  [unwired: 9 in]
          n34 = Tick Count (ms)() -> (millisecond timer value=w98:u32)
          n35 = Subtract(x=w98, y=w99) -> (x-y=w97:u32)
          n36 = Less?(x=w97, y=u32 3000) -> (x < y?=w95:bool)
          n37 = Unbundle(w91) -> ("code"=w90:i32)  [unwired: 2 out]
          n38 = Or(x=w91, y=w95) -> (x .or. y?=w100:bool)
          n39 = call <vilib>:"WPI_UtilitiesFRC Build Error.vi"("error code"=w90, "chain levels to remove (1)"=0) -> ()  [unwired: 3 in, 11 out]
        }
      }
      frame "Reef Align" {
        (unwired) dbl[] [-1.0, -1.0, -1.0, -1.0, -1.0, -60.0, 0.0, 60.0, 120.0, 180.0, 240.0, -1.0, -1.0, -1.0, -1.0, -1.0, 60.0, 0.0, -60.0, -120.0, -180.0, -240.0]
        # "TODO: add in for astra"
        # "x"
        # "y"
        # "th"
        n40 = Quotient & Remainder(x=w111, y=i8 2) -> (x-y*floor(x/y)=w109:i32)  [unwired: 1 out]
        n41 = global read "Robot Global Data.vi" "Robot Mode"() -> (w114:T27)
        n42 = Equal To 0?(x=w109) -> (x = 0?=w108:bool)
        n43 = Equal?(x=w114, y=WPI_DriverStationRobotMode2."Autonomous Enabled") -> (x = y?=w112:bool)
        n44 = Select(t="Even_Tags", s=w108, f="Odd_Tags") -> (s? t:f=w104:string)
        n45 = Select(t=w104, s=w112, f="All_Tags") -> (s? t:f=w102:string)
        n46 = call-poly <vilib>:"NT Write Value.vi"("value"=w102, "name"="limelight_PipelineName") -> ("error out"=w101:errorcluster)  [unwired: 9 in]
        n47 = call-poly <vilib>:"NT Read Value.vi"("error in"=w101, "name"="/limelight-astra/botpose_targetspace") -> ("value"=w138:dbl[])  [unwired: 7 in, 2 out]
        n48 = call-poly <vilib>:"NT Read Value.vi"("error in"=w101, "name"="/limelight/botpose_targetspace") -> ("value"=w135:dbl[])  [unwired: 7 in, 2 out]
        n49 = call-poly <vilib>:"NT Read Value.vi"("error in"=w101, "name"="/limelight/tid") -> ("value"=w141:dbl)  [unwired: 7 in, 2 out]
        n50 = call-poly <vilib>:"NT Read Value.vi"("error in"=w101, "name"="/limelight/tid") -> ("value"=w144:dbl)  [unwired: 7 in, 2 out]
        n51 = Index Array(array=w135, index #1=0 ("index"), index #2=2 ("index"), index #3=4 ("index")) -> (element #1=w126:dbl, element #2=w125:dbl, element #3=w124:dbl)
        n52 = Index Array(array=w138, index #1=0 ("index"), index #2=2 ("index"), index #3=4 ("index")) -> (element #1=w131:dbl, element #2=w130:dbl, element #3=w129:dbl)
        n53 = disable-structure shown="Disabled" {
          disable-tunnel: w131 -> [w154 _]
          disable-tunnel: w126 -> [w153 _]
          frame Disabled {
            n54 = Bundle("Numeric"=w154, "Numeric"=w153) -> (→"Waveform Chart":cluster{"Numeric":dbl, "Numeric":dbl})  [unwired: 1 in]
          }
          frame Enabled {
          }
        }
        n55 = Less Or Equal To 0?(x=w141) -> (x <= 0?=w145:bool)
        n56 = Less Or Equal To 0?(x=w144) -> (x <= 0?=w121:bool)
        n57 = Not And(1:w145, 2:w121) -> (0:w146:bool)
        n58 = Select(t=w144, s=w145, f=w141) -> (s? t:f=w115:dbl)
        n59 = Decrement(x=w115) -> (x-1=w118:dbl)
        n60 = Index Array(array=dbl[] [-1.0, -1.0, -1.0, -1.0, -1.0, -60.0, 0.0, 60.0, 120.0, 180.0, -120.0, -1.0, -1.0, -1.0, -1.0, -1.0, 60.0, 0.0, -60.0, -120.0, -180.0, -240.0] ("Array"), index=w118) -> (element=w116:dbl)
        n61 = disable-structure shown="Enabled" {
          disable-tunnel: [w216 w324] -> w152
          disable-tunnel: w151 -> [w196 w326]
          disable-tunnel: w150 -> [w186 w309]
          disable-tunnel: w149 -> [w185 _]
          disable-tunnel: [w184 _] -> w148
          disable-tunnel: w147 -> [w183 _]
          disable-tunnel: w146 -> [w178 _]
          disable-tunnel: w116 -> [w177 w311]
          disable-tunnel: w145 -> [w176 _]
          disable-tunnel: w144 -> [w175 _]
          disable-tunnel: w138 -> [w174 w354]
          disable-tunnel: w135 -> [w173 w353]
          disable-tunnel: [w170 _] -> w134
          disable-tunnel: w131 -> [_ _]
          disable-tunnel: w130 -> [_ _]
          disable-tunnel: w129 -> [_ _]
          disable-tunnel: w126 -> [w165 _]
          disable-tunnel: w125 -> [w164 _]
          disable-tunnel: w124 -> [w163 _]
          disable-tunnel: "Left X Setpoint" -> [w157 w314]
          disable-tunnel: "Right X Setpoint" -> [w156 w355]
          disable-tunnel: w121 -> [_ w323]
          disable-tunnel: w120 -> [_ w327]
          disable-tunnel: w119 -> [_ w325]
          disable-tunnel: w115 -> [_ w310]
          frame Disabled {
            # "negate removed"
            # "removed negate"
            # "-0.6041666667"
            # "distance from center to limelight"
            # "meters to ft"
            # "0 is left and right, 2 is front and back"
            n62 = Not(x=w176) -> (.not. x?=w166:bool)
            n63 = Select(t=w174, s=w166, f=w173) -> (s? t:f=w179:dbl[])
            n64 = Unbundle By Name(w196) -> ("Pigeon2"=w210:T19)
            n65 = Decrement(x=w175) -> (x-1=w200:dbl)
            n66 = Bundle("Left X Setpoint"=w157, "Left Y Setpoint"="Left Y Setpoint") -> (w189:T34)  [unwired: 1 in]
            n67 = Bundle("Right X Setpoint"=w156, "Right Y Setpoint"="Right Y Setpoint") -> (w187:T35)  [unwired: 1 in]
            n68 = Index Array(array=dbl[] [-1.0, -1.0, -1.0, -1.0, -1.0, -60.0, 0.0, 60.0, 120.0, 180.0, 240.0, -1.0, -1.0, -1.0, -1.0, -1.0, 60.0, 0.0, -60.0, -120.0, -180.0, -240.0], index=w200) -> (element=w199:dbl)
            n69 = call "Generate Trajectory for Alignment.vi"("th"=w164, "y"=w163, "x"=w165) -> ("Trajectory Data Out"=w162:T2)  [unwired: 8 in]
            "Trajectory Data Compare" <- w162
            n70 = call-poly <vilib>:"CTRE_Phoenix_Pigeon2_GetStatus.vi"("PigeonIMUDevRef"=w210) -> ("Yaw Pitch Roll"=w211:cluster{"Yaw":dbl, "Pitch":dbl, "Roll":dbl})  [unwired: 8 in, 2 out]
            n71 = Select(t=w189, s=w186, f=w187) -> (s? t:f=w188:T35)
            n72 = Unbundle(w211) -> ("Yaw"=w202:dbl)  [unwired: 2 out]
            n73 = Add(x=180.0, y=w199) -> (x+y=w182:dbl)
            n74 = Subtract(x=w202, y=w182) -> (x-y=w203:dbl)
            n75 = Multiply(x=w179, y=3.28083 ("x")) -> (x*y=w213:dbl[])
            n76 = Unbundle(w188) -> ("Right X Setpoint"=w168:dbl)  [unwired: 1 out]
            n77 = Index Array(array=w162, index=0) -> (element=w160:T36)
            n78 = expression code="(x/180.0)*pi" "degrees to radians"(w203) -> (w209:dbl)
            n79 = Unbundle By Name(w160) -> ("Traj Vel Points"=w159:T37)
            n80 = Index Array(array=w213, index=0) -> (element=w204:dbl)
            n81 = Sine(x=w209) -> (sin(x)=w208:dbl)
            n82 = Not Equal To 0?(x=w204) -> (x != 0?=w205:bool)
            n83 = for {
              tunnel: w159 -> [w218] mode=indexing
              tunnel: [w217] -> w158 mode=indexing
              n84 = Unbundle By Name(w218) -> ("V"=w217:dbl)
            }
            "Trajectory Velocity" <- w158
            n85 = Multiply(x=w208, y=0.168275) -> (x*y=w206:dbl)
            n86 = Add(x=w206, y=w204) -> (x+y=w167:dbl)
            n87 = Select(t=w167, s=w205, f=0.0) -> (s? t:f=w194:dbl)
            n88 = Unbundle By Name("Deadband") -> ("X (ft)"=w195:dbl)
            n89 = call "Align Velocity.vi"("Period"="Period", "Translational Setpoints"=w168, "AprilTag Pos"=w194, "Deadband"=w195, "Velocity Max"="Velocity Max", "Acceleration Max"="Acceleration Max") -> ("At Setpoint?"=w172:bool, "Array size"=w190:i32, "Velocity values"=w169:dbl[])  [unwired: 1 in]
            n90 = Not(x=w172) -> (.not. x?=w171:bool)
            n91 = case shown="True" w178 {
              tunnel: [FALSE w233] -> w216
              tunnel: w169 -> [_ w242]
              tunnel: w171 -> [_ w241]
              tunnel: w196 -> [w223 w234]
              tunnel: "Period" -> [_ w230]
              tunnel: w177 -> [_ w231]
              tunnel: w190 -> [_ w240]
              tunnel: w185 -> [w224 _]
              tunnel: [20.0 -1.0] -> w184
              tunnel: w183 -> [_ w235]
              tunnel: w168 -> [_ w232]
              tunnel: ["nah we cool" "yeah :("] -> w170
              tunnel: w169 -> [_ w228]
              frame False {
                n92 = call "NEO Swerve Drive.vi"("Drive Conditions"=cluster{"Field Centric":bool, "Reef Align":bool} {"Field Centric"=TRUE, "Reef Align"=FALSE}, "Robot Velocities"=w224, "Swerve Drive"=w223) -> ()  [unwired: 8 in, 1 out]
              }
              frame True {
                n93 = call "Trapezoid Align.vi"("Angle Align"=w235, "Motors"=w234, "Array size"=w240, "Period"=w230, "Go Up?"="Go Up?", "value"=w231, "Boolean 3"=w241, "Velocity values"=w242) -> ("Boolean 2"=w238:bool, "Boolean"=w237:bool)  [unwired: 2 in]
                n94 = And(x="PID enabled", y=w238) -> (x .and. y?=w227:bool)
                n95 = case shown="True" w227 {
                  tunnel: [FALSE w249] -> w236
                  tunnel: w235 -> [_ w248]
                  tunnel: w234 -> [_ w247]
                  tunnel: w232 -> [_ w246]
                  tunnel: w230 -> [_ w245]
                  tunnel: w231 -> [_ w244]
                  frame False {
                  }
                  frame True {
                    n96 = node-c288(w245) -> (w251:T28)
                    n97 = timed-loop {
                      timing: w251 -> [_]
                      timing-out: [_] -> w250
                      tunnel: [w290] -> w249
                      tunnel: w248 -> [w281]
                      tunnel: w247 -> [w280]
                      tunnel: w246 -> [w276]
                      tunnel: w244 -> [w258]
                      stop <- w290 stop-if-true
                      w270 = 3.28083 ("x")
                      n98 = node-c288() -> ()  [unwired: 1 in, 1 out]
                      n99 = call-poly <vilib>:"NT Read Value.vi"("name"="/limelight-four/botpose_targetspace") -> ("value"=w255:dbl[])  [unwired: 8 in, 2 out]
                      n100 = call-poly <vilib>:"NT Read Value.vi"("name"="/limelight-four/botpose_targetspace") -> ("value"=w256:dbl[])  [unwired: 8 in, 2 out]
                      n101 = global read "Robot Global Data.vi" "Robot Velocities"() -> (w287:T11)
                      n102 = call-poly <vilib>:"NT Read Value.vi"("name"="/limelight-four/tid") -> ("value"=w274:dbl)  [unwired: 8 in, 2 out]
                      n103 = call-poly <vilib>:"NT Read Value.vi"("name"="/limelight-astra/tid") -> ("value"=w259:dbl)  [unwired: 8 in, 2 out]
                      n104 = Unbundle By Name(w287) -> ("Y Velocity"=w285:dbl)
                      n105 = Equal?(x=w274, y=w258) -> (x = y?=w253:bool)
                      n106 = Equal?(x=w259, y=w258) -> (x = y?=w260:bool)
                      n107 = Select(t=w256, s=w253, f=w255) -> (s? t:f=w254:dbl[])
                      n108 = Index Array(array=w254, index #1=0 ("index"), index #2=2 ("index")) -> (element #1=w277:dbl, element #2=w271:dbl)
                      n109 = Multiply(x=w277, y=w270) -> (x*y=w273:dbl)
                      n110 = Multiply(x=w270, y=w271) -> (x*y=w269:dbl)
                      n111 = Multiply(x=w269, y="Int per ft") -> (x*y=w267:dbl)
                      n112 = Absolute Value(x=w267) -> (abs(x)=w266:dbl)
                      n113 = Round Toward -Infinity(1:w266) -> (0:w265:dbl)
                      n114 = Add(x=w265, y=4.0) -> (x+y=w263:dbl)
                      n115 = call <vilib>:"Median Filter PtByPt.vi"("rank"=w263, "x"=w273) -> ("Filtered x"=w252:dbl)  [unwired: 2 in, 1 out]
                      n116 = Bundle("Filtered x"=w252, "Right X Setpoint"=w276) -> (→"Waveform Chart":T38)  [unwired: 1 in]
                      n117 = Or(x=w253, y=w260) -> (x .or. y?=w261:bool)
                      n118 = case shown="True" w261 {
                        tunnel: [0.0 ("output") w297] -> w278
                        tunnel: w276 -> [_ w296]
                        tunnel: w252 -> [_ w294]
                        frame False {
                        }
                        frame True {
                          n119 = call <vilib>:"Parallel PID (DBL).vi"("output range"=cluster{"high":dbl, "low":dbl} {"high"=10.0, "low"=-10.0}, "PID gains"="PID gains", "process variable"=w294, "setpoint"=w296) -> ("output"=w297:dbl)  [unwired: 4 in, 3 out]
                        }
                      }
                      "PID Out" <- w278
                      n120 = Bundle("output"=w278, "Y Velocity"=w285, 0.0) -> (w284:cluster{"output":dbl, "Y Velocity":dbl, dbl})  [unwired: 1 in]
                      n121 = call "NEO Swerve Drive.vi"("Angle Align"=w281, "Operation"="Operation", "Offset from 0"=w258, "Drive Conditions"=cluster{"Field Centric":bool, "Reef Align":bool} {"Field Centric"=TRUE, "Reef Align"=TRUE}, "Robot Velocities"=w284, "Swerve Drive"=w280) -> ()  [unwired: 5 in, 1 out]
                      n122 = global read "Robot Global Data.vi" "Aligning?"() -> (w291:bool)
                      n123 = node-c288() -> ()  [unwired: 1 in, 1 out]
                      n124 = Not(x=w291) -> (.not. x?=w290:bool)
                    }
                    n125 = node-c288(w250) -> ()  [unwired: 1 out]
                  }
                }
                n126 = Or(x=w236, y=w237) -> (x .or. y?=w233:bool)
                "Trapezoid Profile" <- w228
              }
            }
          }
          frame Enabled {
            # "TODO: check?"
            # "Limelight 4 can't see?"
            # "TODO:  fix using limelight four only"
            n127 = Select(t=w354, s=w323, f=w353) -> (s? t:f=w352:dbl[])
            n128 = Index Array(array=w352, index #1=0 ("index"), index #2=2 ("index"), index #3=4 ("index")) -> (element #1=w316:dbl, element #2=w320:dbl, element #3=w348:dbl)
            n129 = Multiply(x=w320, y=3.28084) -> (x*y=w319:dbl)
            n130 = disable-structure shown="Enabled" {
              disable-tunnel: w323 -> [w373 w374]
              disable-tunnel: [w370 w375] -> w322
              disable-tunnel: w319 -> [w368 w375]
              disable-tunnel: [_ w374] -> w313
              frame Disabled {
                # "this \"subtraction\" always changes just\nthe y-component, which doesn't account\nfor rotation"
                n131 = Select(t=1.416667 ("x"), s=w373, f=1.166667) -> (s? t:f=w369:dbl)
                n132 = Add(x=w368, y=w369) -> (x+y=w370:dbl)
              }
              frame Enabled {
              }
            }
            n133 = Multiply(x=3.28084 ("y"), y=w316) -> (x*y=w315:dbl)
            n134 = disable-structure shown="Enabled" {
              disable-tunnel: w313 -> [w366 _]
              disable-tunnel: [w363 "Y Setpoint"] -> w312
              frame Disabled {
                n135 = Select(t=-1.416667 ("x"), s=w366, f=-1.166667) -> (s? t:f=w363:dbl)
              }
              frame Enabled {
              }
            }
            n136 = Select(t=w314, s=w309, f=w355) -> (s? t:f=w347:dbl)
            n137 = Bundle("Right X Setpoint"=w347, "Y Setpoint"=w312, 0.0) -> (w345:T39)  [unwired: 1 in]
            n138 = Select(t="Left PID Setpoint", s=w309, f="Right PID Setpoint") -> (s? t:f=w306:dbl)
            n139 = call "Generate Trajectory for Alignment.vi"("Setpoints"=w345, "th"=w348, "y"=w322, "x"=w315) -> ("Trajectory Data Out"=w361:T2)  [unwired: 7 in]
            "Trajectory Data Out" <- w361
            n140 = Index Array(array=w361) -> (element=w360:T36)  [unwired: 1 in]
            n141 = Unbundle By Name(w360) -> ("Traj Vel Points"=w357:T37, "Traj Pos Points"=w358:cluster{"x":dbl, "y":dbl, "th":dbl}[])
            n142 = for {
              tunnel: w357 -> [w402] mode=indexing
              tunnel: [w401] -> w304 mode=indexing
              tunnel: [w399] -> w344 mode=indexing
              tunnel: [w400] -> w339 mode=indexing
              tunnel: [w396] -> w341 mode=indexing
              tunnel: [w399] -> w343 mode=indexing
              tunnel: [w398] -> w331 mode=indexing
              n143 = Unbundle By Name(w402) -> ("V vector.x"=w399:dbl, "V vector.y"=w397:dbl, "Omega"=w400:dbl, "V"=w398:dbl)
              n144 = Negate(x=w397) -> (-x=w396:dbl)
              n145 = Bundle("x"=w399, w396, "Omega"=w400) -> (w401:cluster{"x":dbl, dbl, "Omega":dbl})  [unwired: 1 in]
            }
            "Enabled X Velocity" <- w344
            "Enabled Omega" <- w339
            "Enabled Y Velocity" <- w341
            "Enabled VMag" <- w331
            n146 = Array Size(array=w304) -> (size(s)=w305:i32)
            n147 = case shown="..3" w305 {
              frame Default {
              }
              frame ..3 {
              }
            }
            n148 = Add Array Elements(numeric array=w331) -> (sum=w330:dbl)
            n149 = Add Array Elements(numeric array=w341) -> (sum=w340:dbl)
            n150 = Multiply(x=w330, y=0.02) -> (x*y=→"VMag Sum":dbl)
            n151 = Multiply(x=w340, y=0.02) -> (x*y=→"Sum Y":dbl)
            n152 = Add Array Elements(numeric array=w343) -> (sum=w342:dbl)
            n153 = Multiply(x=0.02, y=w342) -> (x*y=→"Sum X":dbl)
            n154 = Bundle By Name(cluster=T31 {"Auto Velocities"=[], "Auto Positions"=[], "Auto Commands"=[], "Zero Velocity?"=[]} ("Auto Data"), "Auto Velocities"=w304, "Auto Positions"=w358) -> (w356:T31)
            n155 = Add Array Elements(numeric array=w339) -> (sum=w336:dbl)
            n156 = Multiply(x=w336, y=0.02) -> (x*y=→"Sum Angle":dbl)
            n157 = disable-structure shown="Enabled" {
              disable-tunnel: enum16{"Start", "Wait"}."Start" ("Synchronization") -> [w377 _]
              disable-tunnel: w356 -> [w376 w384]
              disable-tunnel: w327 -> [_ w386]
              disable-tunnel: w326 -> [_ w385]
              disable-tunnel: w325 -> [_ w383]
              disable-tunnel: [_ w382] -> w324
              disable-tunnel: "Freeze Align?" -> [_ w381]
              disable-tunnel: w311 -> [_ w380]
              disable-tunnel: w310 -> [_ w379]
              disable-tunnel: w306 -> [_ w378]
              frame Disabled {
                n158 = call "Play Path.vi"("Synchronization"=w377, "Auto Data"=w376) -> ()  [unwired: 9 in, 1 out]
              }
              frame Enabled {
                n159 = case shown="False" w381 {
                  tunnel: w386 -> [w394 _]
                  tunnel: w385 -> [w393 _]
                  tunnel: w384 -> [w392 _]
                  tunnel: w383 -> [w391 _]
                  tunnel: [w390 TRUE ("Auto Done?")] -> w382
                  tunnel: w380 -> [w389 _]
                  tunnel: w379 -> [w388 _]
                  tunnel: w378 -> [w387 _]
                  frame False {
                    n160 = call "Reef Align Play Path.vi"("PID setpoint"=w387, "Tag ID"=w388, "PID Constants"=w394, "Operation"=w391, "Auto Data"=w392, "Motors"=w393, "AprilTag Offset"=w389) -> ("Auto Done?"=w390:bool)  [unwired: 4 in]
                  }
                  frame True {
                  }
                }
              }
            }
          }
        }
        "Weird Aligning Code?" <- w134
      }
    }
    n161 = disable-structure shown="Enabled" {
      disable-tunnel: w24 -> [w37 _]
      disable-tunnel: w23 -> [w34 _]
      frame Disabled {
        n162 = call "NEO Get Sensor Values.vi"("Swerve Motors"=w34) -> ("Steer Angles (degrees)"=w35:T9, "Drive Velocities (ft/s)"=w36:T9)  [unwired: 9 in]
        n163 = call "Swerve Drive Visuals.vi"("Steer Angles (degrees)"=w35, "Drive Velocities (ft/s)"=w36, "Pod Setpoints (ft/s and deg)"=w37) -> ("Swerve Visualizer"=→"Swerve Visualizer":cluster{dbl[], dbl[]}[], "Pod Comparisons (Diff -> Setpoint - Actual)"=→"Pod Comparisons (Diff -> Setpoint - Actual)":T8)  [unwired: 7 in]
      }
      frame Enabled {
      }
    }
    n164 = call "Drive Check for New Command.vi"("input cluster"=w16, "Wait time (ms)"=w31, "Finished?"=w30) -> ("Completion"=w21:T23, "Subsystem Name"=w28:string, "Current Command"=w20:T10, "Initial Trace String"=w29:string, "Next Command"=w25:T40)  [unwired: 4 in]
    n165 = case shown="\"Successful\", \"Aborted\"" w21 {
      selector: w21 -> [_ w403]
      tunnel: w29 -> [_ w410]
      tunnel: w20 -> [_ w411]
      tunnel: w28 -> [_ w409]
      frame "Incomplete", Default {
        # "Continuing current command"
      }
      frame "Successful", "Aborted" {
        # "Report and setup for next command"
        n166 = Unbundle By Name(w411) -> ("Robot Velocities.X Velocity"=w407:dbl, "Robot Velocities.Y Velocity"=w408:dbl, "Robot Velocities.Rotational \nVelocity"=w404:dbl)
        n167 = Format Into String(format string="Vx %.1f, Vy %.1f, W %f", initial string=w410, w407, w408, w404) -> (resulting string=w405:string)  [unwired: 1 in, 1 out]
        "Current\nCmd" <- w405
        n168 = call <vilib>:"Trace Results.vi"("Status of previous command"=w403, "Description"=w405, "Subsystem"=w409) -> ()  [unwired: 9 in]
      }
    }
  }
